vi "BRig_dataMTrig_warmup_struct.vi"() -> (2 "output_warmup_struct":i32)   [LabVIEW 2014]
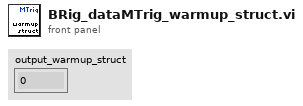
[diagram p1: front panel]
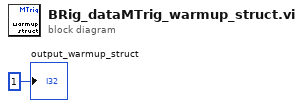
[diagram p0: block diagram]
diagram:
  "output_warmup_struct" <- 1 ("output_iBlock")
